vi "sub_3x3_indexes.vi"() -> (3 "3x3 matrix indexes":cluster{"row":i32, "col":i32}[](array[cluster]))   [LabVIEW 2018]
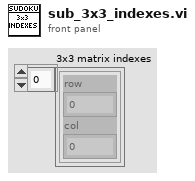
[diagram p1: front panel]
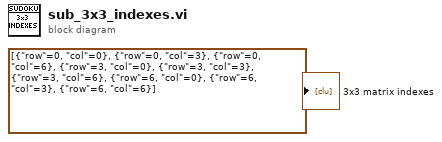
[diagram p0: block diagram]
diagram:
  "3x3 matrix indexes" <- cluster{"row":i32, "col":i32}[] [{"row"=0, "col"=0}, {"row"=0, "col"=3}, {"row"=0, "col"=6}, {"row"=3, "col"=0}, {"row"=3, "col"=3}, {"row"=3, "col"=6}, {"row"=6, "col"=0}, {"row"=6, "col"=3}, {"row"=6, "col"=6}]
